vi "read_language_file.vi"(11 "Text File":path) -> (3 "gui_strings":string[](array[string]))   [LabVIEW 2013]
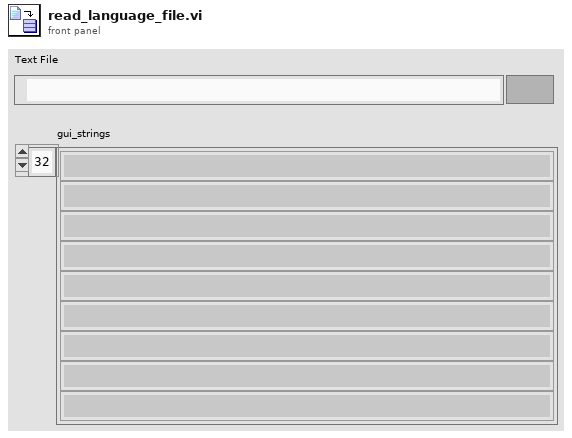
[diagram p1: front panel]
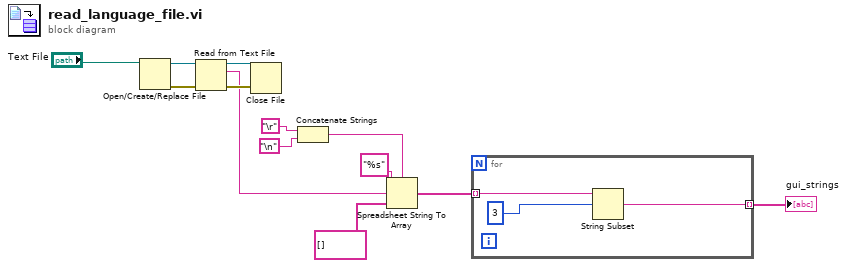
[diagram p0: block diagram]
diagram:
  n1 = Open/Create/Replace File(file path (use dialog)="Text File") -> (refnum out=w11:refnum<file>, error out=w12:errorcluster)  [unwired: 5 in, 1 out]
  n2 = Read from Text File(file (use dialog)=w11, error in=w12) -> (refnum out=w10:refnum<file>, text=w6:string, error out=w9:errorcluster)  [unwired: 2 in, 1 out]
  n3 = Close File(refnum=w10, error in=w9) -> ()  [unwired: 2 out]
  n4 = Concatenate Strings("\r", "\n") -> (w1:string)
  n5 = Spreadsheet String To Array(delimiter (Tab)=w1, format string="%s", spreadsheet string=w6, array type (2D Dbl)=string[] []) -> (array=w5:string[])
  n6 = for {
    tunnel: w5 -> [w16] mode=indexing
    tunnel: [w14] -> w4 mode=indexing
    n7 = String Subset(string=w16, offset (0)=3) -> (substring=w14:string)  [unwired: 1 in]
  }
  "gui_strings" <- w4
